vi "I2C LCD - Write Byte.vi"(6 "BL":bool, 7 "RS":bool, 8 "error in (no error)":errorcluster, 9 "Slave Address (7-bit)":u8, 10 "Numeric":u8, 11 "I2C Ref":T1) -> (0 "error out":errorcluster, 3 "I2C Ref Out":T1)   [LabVIEW 2017]
uses:
  <vilib>/myRIO/Instrument Drivers/Onboard IO/I2C/typedefs/I2C Reference.ctl
  <vilib>/myRIO/Common/Instrument Driver Framework/Utilities/typedefs/myRIO Generic Hardware Reference.ctl
  <vilib>/myRIO/Common/Instrument Driver Framework/Utilities/typedefs/Hardware Version Enum.ctl
  <vilib>/myRIO/Common/Instrument Driver Framework/Utilities/typedefs/myRIO v1.0 Reference.ctl
  <vilib>/myRIO/Common/Instrument Driver Framework/Utilities/typedefs/Generic FPGA Reference.ctl
  <vilib>/myRIO/Common/Instrument Driver Framework/myRIO v1.0/I2C/typedefs/I2C Channels Enum.ctl
  <vilib>/myRIO/Instrument Drivers/Onboard IO/I2C/typedefs/I2C Configuration.ctl
  <vilib>/myRIO/Instrument Drivers/Onboard IO/I2C/typedefs/I2C Transfer Rate.ctl
  <vilib>/Utility/error.llb/Error Cluster From Error Code.vi
  <vilib>/myRIO/Common/Instrument Driver Framework/myRIO v1.0/I2C/vis/myRIO v1.0 Write I2C.vi
  <vilib>/myRIO/Instrument Drivers/Onboard IO/I2C/I2C.lvlib
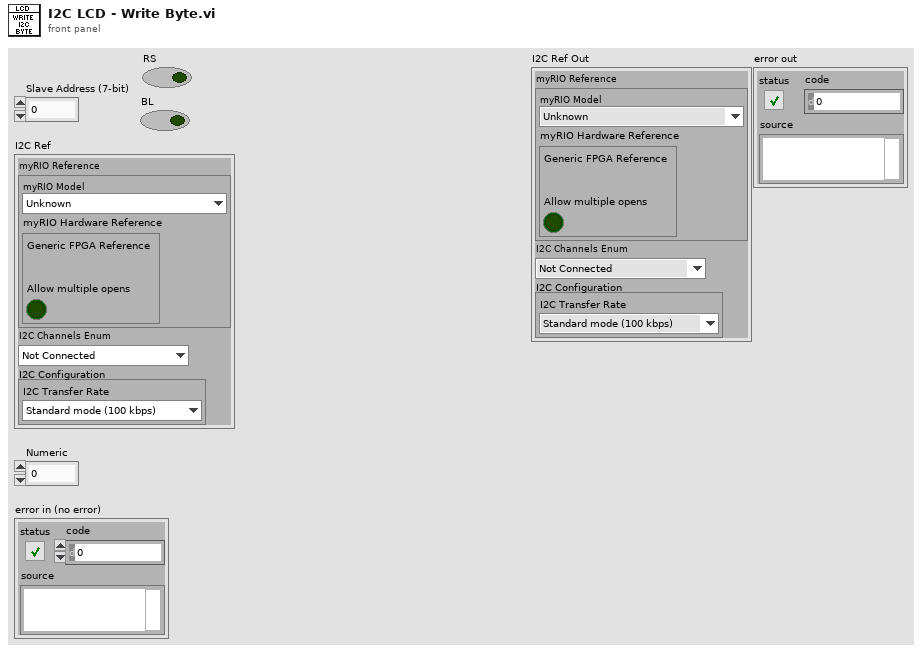
[diagram p1: front panel]
types:
  T1 = typedef "I2C.lvlib/I2C Reference.ctl" = cluster{"myRIO Reference":T2, "I2C Channels Enum":T6, "I2C Configuration":T7}
  T2 = typedef "myRIO Generic Hardware Reference.ctl" = cluster{"myRIO Model":T3, "myRIO Hardware Reference":T4}
  T3 = typedef "Hardware Version Enum.ctl" = enum16{"Unknown", "myRIO-1900", "myRIO-1950", "roboRIO", "NI ELVIS RIO CM"}
  T4 = typedef "myRIO v1.0 Reference.ctl" = cluster{"Generic FPGA Reference":T5, "Allow multiple opens":bool}
  T5 = typedef "Generic FPGA Reference.ctl" = refnum<k20>
  T6 = typedef "I2C Channels Enum.ctl" = enum16{"Not Connected", "A/I2C", "B/I2C", "I2C/I2C"}
  T7 = typedef "I2C.lvlib/I2C Configuration.ctl" = cluster{"I2C Transfer Rate":T8}
  T8 = typedef "I2C.lvlib/I2C Transfer Rate.ctl" = enum16{"Standard mode (100 kbps)", "Fast mode (400 kbps)"}
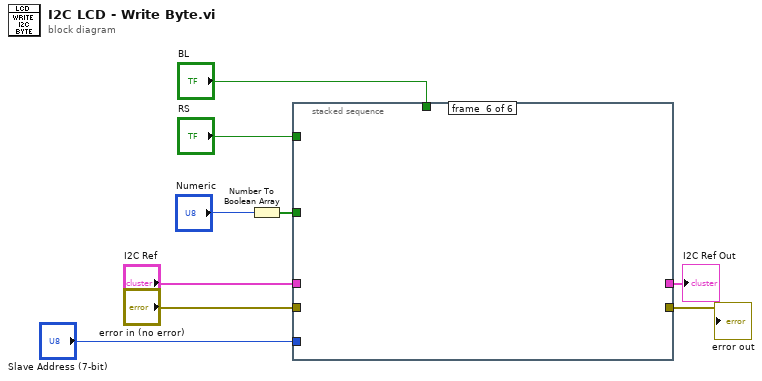
[diagram p0: block diagram]
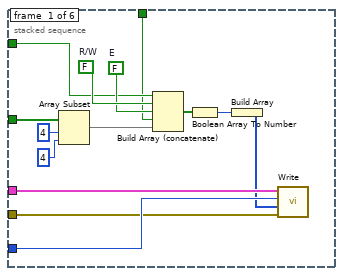
[diagram p2: hidden frame]
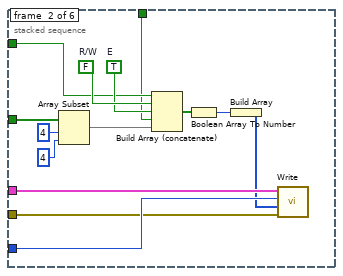
[diagram p3: hidden frame]
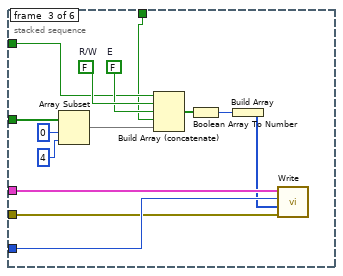
[diagram p4: hidden frame]
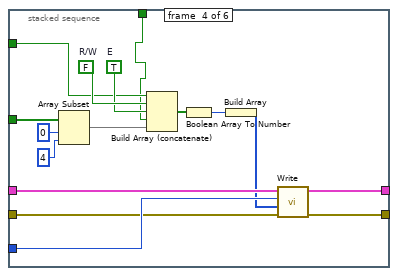
[diagram p5: hidden frame]
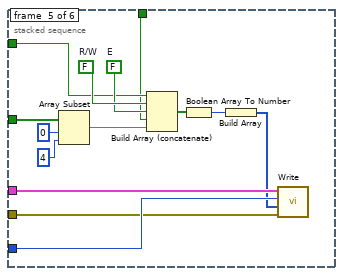
[diagram p6: hidden frame]
diagram:
  n1 = Number To Boolean Array(number="Numeric") -> (Boolean array=w7:bool[])
  n2 = stacked-sequence {
    tunnel: "Slave Address (7-bit)" -> [w23 w37 w51 w67 w81 _]
    tunnel: w7 -> [w22 w36 w50 w66 w80 _]
    tunnel: "I2C Ref" -> [w15 w29 w43 w59 w73 _]
    tunnel: "error in (no error)" -> [w14 w28 w42 w58 w72 _]
    tunnel: "RS" -> [w11 w25 w39 w55 w69 _]
    tunnel: [_ _ _ w54 _ _] -> w3
    tunnel: [_ _ _ w53 _ _] -> w2
    tunnel: "BL" -> [w10 w24 w38 w52 w68 _]
    frame #0 {
      w19 = FALSE  # E
      w20 = FALSE  # R/W
      n3 = Array Subset(array=w22, index=u8 4, length=u8 4) -> (w21:bool[])
      n4 = Build Array (concatenate)(w11, w20, w19, w10, w21) -> (w16:bool[])
      n5 = Boolean Array To Number(Boolean array=w16) -> (number=w13:u8)
      n6 = Build Array(w13) -> (w12:u8[])
      n7 = call <vilib>:"Write.vi"("error in (no error)"=w14, "Bytes to Write"=w12, "Slave Address (7-bit)"=w23, "I2C Ref In"=w15) -> ()  [unwired: 6 in, 2 out]
    }
    frame #1 {
      w33 = TRUE  # E
      w34 = FALSE  # R/W
      n8 = Array Subset(array=w36, index=u8 4, length=u8 4) -> (w35:bool[])
      n9 = Build Array (concatenate)(w25, w34, w33, w24, w35) -> (w30:bool[])
      n10 = Boolean Array To Number(Boolean array=w30) -> (number=w27:u8)
      n11 = Build Array(w27) -> (w26:u8[])
      n12 = call <vilib>:"Write.vi"("error in (no error)"=w28, "Bytes to Write"=w26, "Slave Address (7-bit)"=w37, "I2C Ref In"=w29) -> ()  [unwired: 6 in, 2 out]
    }
    frame #2 {
      w47 = FALSE  # E
      w48 = FALSE  # R/W
      n13 = Array Subset(array=w50, index=u8 0, length=u8 4) -> (w49:bool[])
      n14 = Build Array (concatenate)(w39, w48, w47, w38, w49) -> (w44:bool[])
      n15 = Boolean Array To Number(Boolean array=w44) -> (number=w41:u8)
      n16 = Build Array(w41) -> (w40:u8[])
      n17 = call <vilib>:"Write.vi"("error in (no error)"=w42, "Bytes to Write"=w40, "Slave Address (7-bit)"=w51, "I2C Ref In"=w43) -> ()  [unwired: 6 in, 2 out]
    }
    frame #3 {
      w63 = TRUE  # E
      w64 = FALSE  # R/W
      n18 = Array Subset(array=w66, index=u8 0, length=u8 4) -> (w65:bool[])
      n19 = Build Array (concatenate)(w55, w64, w63, w52, w65) -> (w60:bool[])
      n20 = Boolean Array To Number(Boolean array=w60) -> (number=w57:u8)
      n21 = Build Array(w57) -> (w56:u8[])
      n22 = call <vilib>:"Write.vi"("error in (no error)"=w58, "Bytes to Write"=w56, "Slave Address (7-bit)"=w67, "I2C Ref In"=w59) -> ("error out"=w53:errorcluster, "I2C Ref Out"=w54:T1)  [unwired: 6 in]
    }
    frame #4 {
      w77 = FALSE  # E
      w78 = FALSE  # R/W
      n23 = Array Subset(array=w80, index=u8 0, length=u8 4) -> (w79:bool[])
      n24 = Build Array (concatenate)(w69, w78, w77, w68, w79) -> (w74:bool[])
      n25 = Boolean Array To Number(Boolean array=w74) -> (number=w71:u8)
      n26 = Build Array(w71) -> (w70:u8[])
      n27 = call <vilib>:"Write.vi"("error in (no error)"=w72, "Bytes to Write"=w70, "Slave Address (7-bit)"=w81, "I2C Ref In"=w73) -> ()  [unwired: 6 in, 2 out]
    }
    frame #5 {
    }
  }
  "I2C Ref Out" <- w3
  "error out" <- w2
